vi "Doppler_SVM.vi"(7 "PRF1/2":bool=TRUE, 9 "Doppler Params":T1={"Dopp Filter Order"=2, "Window length"=64, "Window Increment"=64, "Start f"=0.05, "lDoppler cutouff"=10.0, "FFT Length"=512, "SlowTime (Hz)"=100.0} {"Start f" format="%0.3f"; "SlowTime (Hz)" format="%0.1f"; "lDoppler cutouff" format="%0.3f"}, 10 "Input Array":csg[][][](array[numeric]), 11 "Header In":T4={"header info"={"Header"="", "Head length"=0}, "A/D info"={"# rf points per line"=0, "# lines per scan"=0, "sample rate MHz"=0, "# A/D bits"=0, "# bytes per A/D"=0, "TGC Flag"=0, "A/D Type"=""}, "Tranducer Info"={"bandwidth"=0.0, "center freq"=0.0, "start freq"=0.0, "ID"=0}, "Scan Info"={"delay"=0.0, "pivot distance"=0.0, "sector scan angle"=0.0, "operator"="", "Scan Mode"="", "location"=""}, "Time/Date Info"={"date"="", "time"=""}, "RF Info"={"RF file name"="", "RF file att"="", "RF cal file name"="", "RF cal file att"=""}, "Patient Info"={"ID"="", "extended ID"="", "age"=0, "sex"="", "previously\nscanned"="", "PSA"=0.0, "LOS"=1, "Ethnicty 2"=3, "Race"=3}, "Tissue Type"={"organ"=0, "disease type"=0, "disease location"=0, "IQ_pts"=0, "RcvBuffer"=0, "RcvFrame"=0, "IQBuff"=0, "IQFrame"=0, "IQPage"=0}, "Votage scaling"={"Digitizer (dB)"=0.0, "Gain (dB)"=0.0, "Atten (dB)"=0.0}, "Comment"="", "Misc Info"={"avg num"=0, "c speed"=0, "Div By or SF zones"=0, "XMIT CHS"=0, "RCV CHS"=0, "Xmit angle"=0.0}, "Therapy Parameters"={"Theraputic Freq (MHz)"=0.1, "Time on (s)"=1.0, "Therapy amplitude (mV)"=50.0, "Lines Before"=20, "Lines After"=80}, "Scan Settings"={"Energy (uJ or V)"=0, "Damp (Ohm) or Fc"=0, "HP Filt (KHz)"=0, "LP Filt (MHz)"=0, "Gain (db)"=0, "prf (kHz)"=0.0, "Distance between\nscan lines (um)"=0, "Distance between\nscan planes (um)"=0, "Scan line gap (um)"=0.0, "Scan plane gap (um)"=0.0}, "Compression Parameters"={"F1 (MHz)"=0.0, "F2 (MHz)"=0.0, "% taper"=0.0, "duration"=0.0}, "Patient Info Xtra"={"First Name"="", "Last Name"="", "Notes"=""}, "ROI Box"=[]} {"Compression Parameters"."% taper" min=50 max=1000 format="%.2f"; "Compression Parameters"."F2 (MHz)" format="%.3f"; "Compression Parameters"."F1 (MHz)" format="%.3f"; "Scan Settings"."prf (kHz)" format="%.2f"; "Therapy Parameters"."Therapy amplitude (mV)" min=50 max=1000 format="%.2f"; "Therapy Parameters"."Time on (s)" format="%.3f"; "Therapy Parameters"."Theraputic Freq (MHz)" format="%.3f"; "Patient Info"."Race" items=["Am Ind or Alaska", "Asian", "Hawaiian, Pac Isl", "Black or Afr Amer", "White", "more than one race", "unknown"]; "Patient Info"."Ethnicty 2" items=["Hispanic", "Non-Hispanic", "unknown"]; "Patient Info"."LOS" items=["1", "2", "3", "4", "5"]; "Patient Info"."PSA" format="%.1f"; "Scan Info"."delay" format="%.2f"; "Scan Info"."pivot distance" format="%.2f"; "Scan Info"."sector scan angle" format="%.2f"; "Tranducer Info"."bandwidth" format="%.2f"; "Tranducer Info"."center freq" format="%.2f"; "Tranducer Info"."start freq" format="%.2f"}) -> (2 "output cluster":T3, 3 "Filtered Output":cdb[][][](array[numeric]))   [LabVIEW 2022 SP3]
uses:
  ViewData/-ReadEye/Header.ctl
  <vilib>/Analysis/Matrix/Datatypes/ComplexMatrix.ctl
  DopplerParams.ctl
  <vilib>/Analysis/7linalg.llb/Complex Conjugate Transpose Matrix.vi
  <vilib>/Analysis/baseanly.llb/Complex A x B.vi
  <vilib>/Analysis/7linalg.llb/Complex Eigenvalues and Vectors.vi
  <vilib>/Analysis/4window.llb/Hamming Window (CDB).vi
  <vilib>/Analysis/2dsp.llb/Complex FFT.vi
  <vilib>/Analysis/baseanly.llb/Scale 1D.vi
  <vilib>/Analysis/4window.llb/AllCosWindow (CDB).vi
  <vilib>/Analysis/NI_AALPro.lvlib
  <vilib>/Analysis/NI_AALBase.lvlib
  <vilib>/Analysis/Matrix/NI_Matrix.lvlib
panel:
  out "Spectro fig":dbl[][](graph)
  out "Sing Value Sum":dbl[](graph)
  out "raw":sgl[][](graph)
  out "Dop Freq":dbl[](graph)
  out "filtered data":dbl[][](graph)
  in  "v? or f":bool
  out "Covariance":dbl[][](graph)
  out "Sing Value Diff Ratio":dbl[](graph)
  out "Sing Values":dbl[](graph)
  in  "GapCutOff":i16
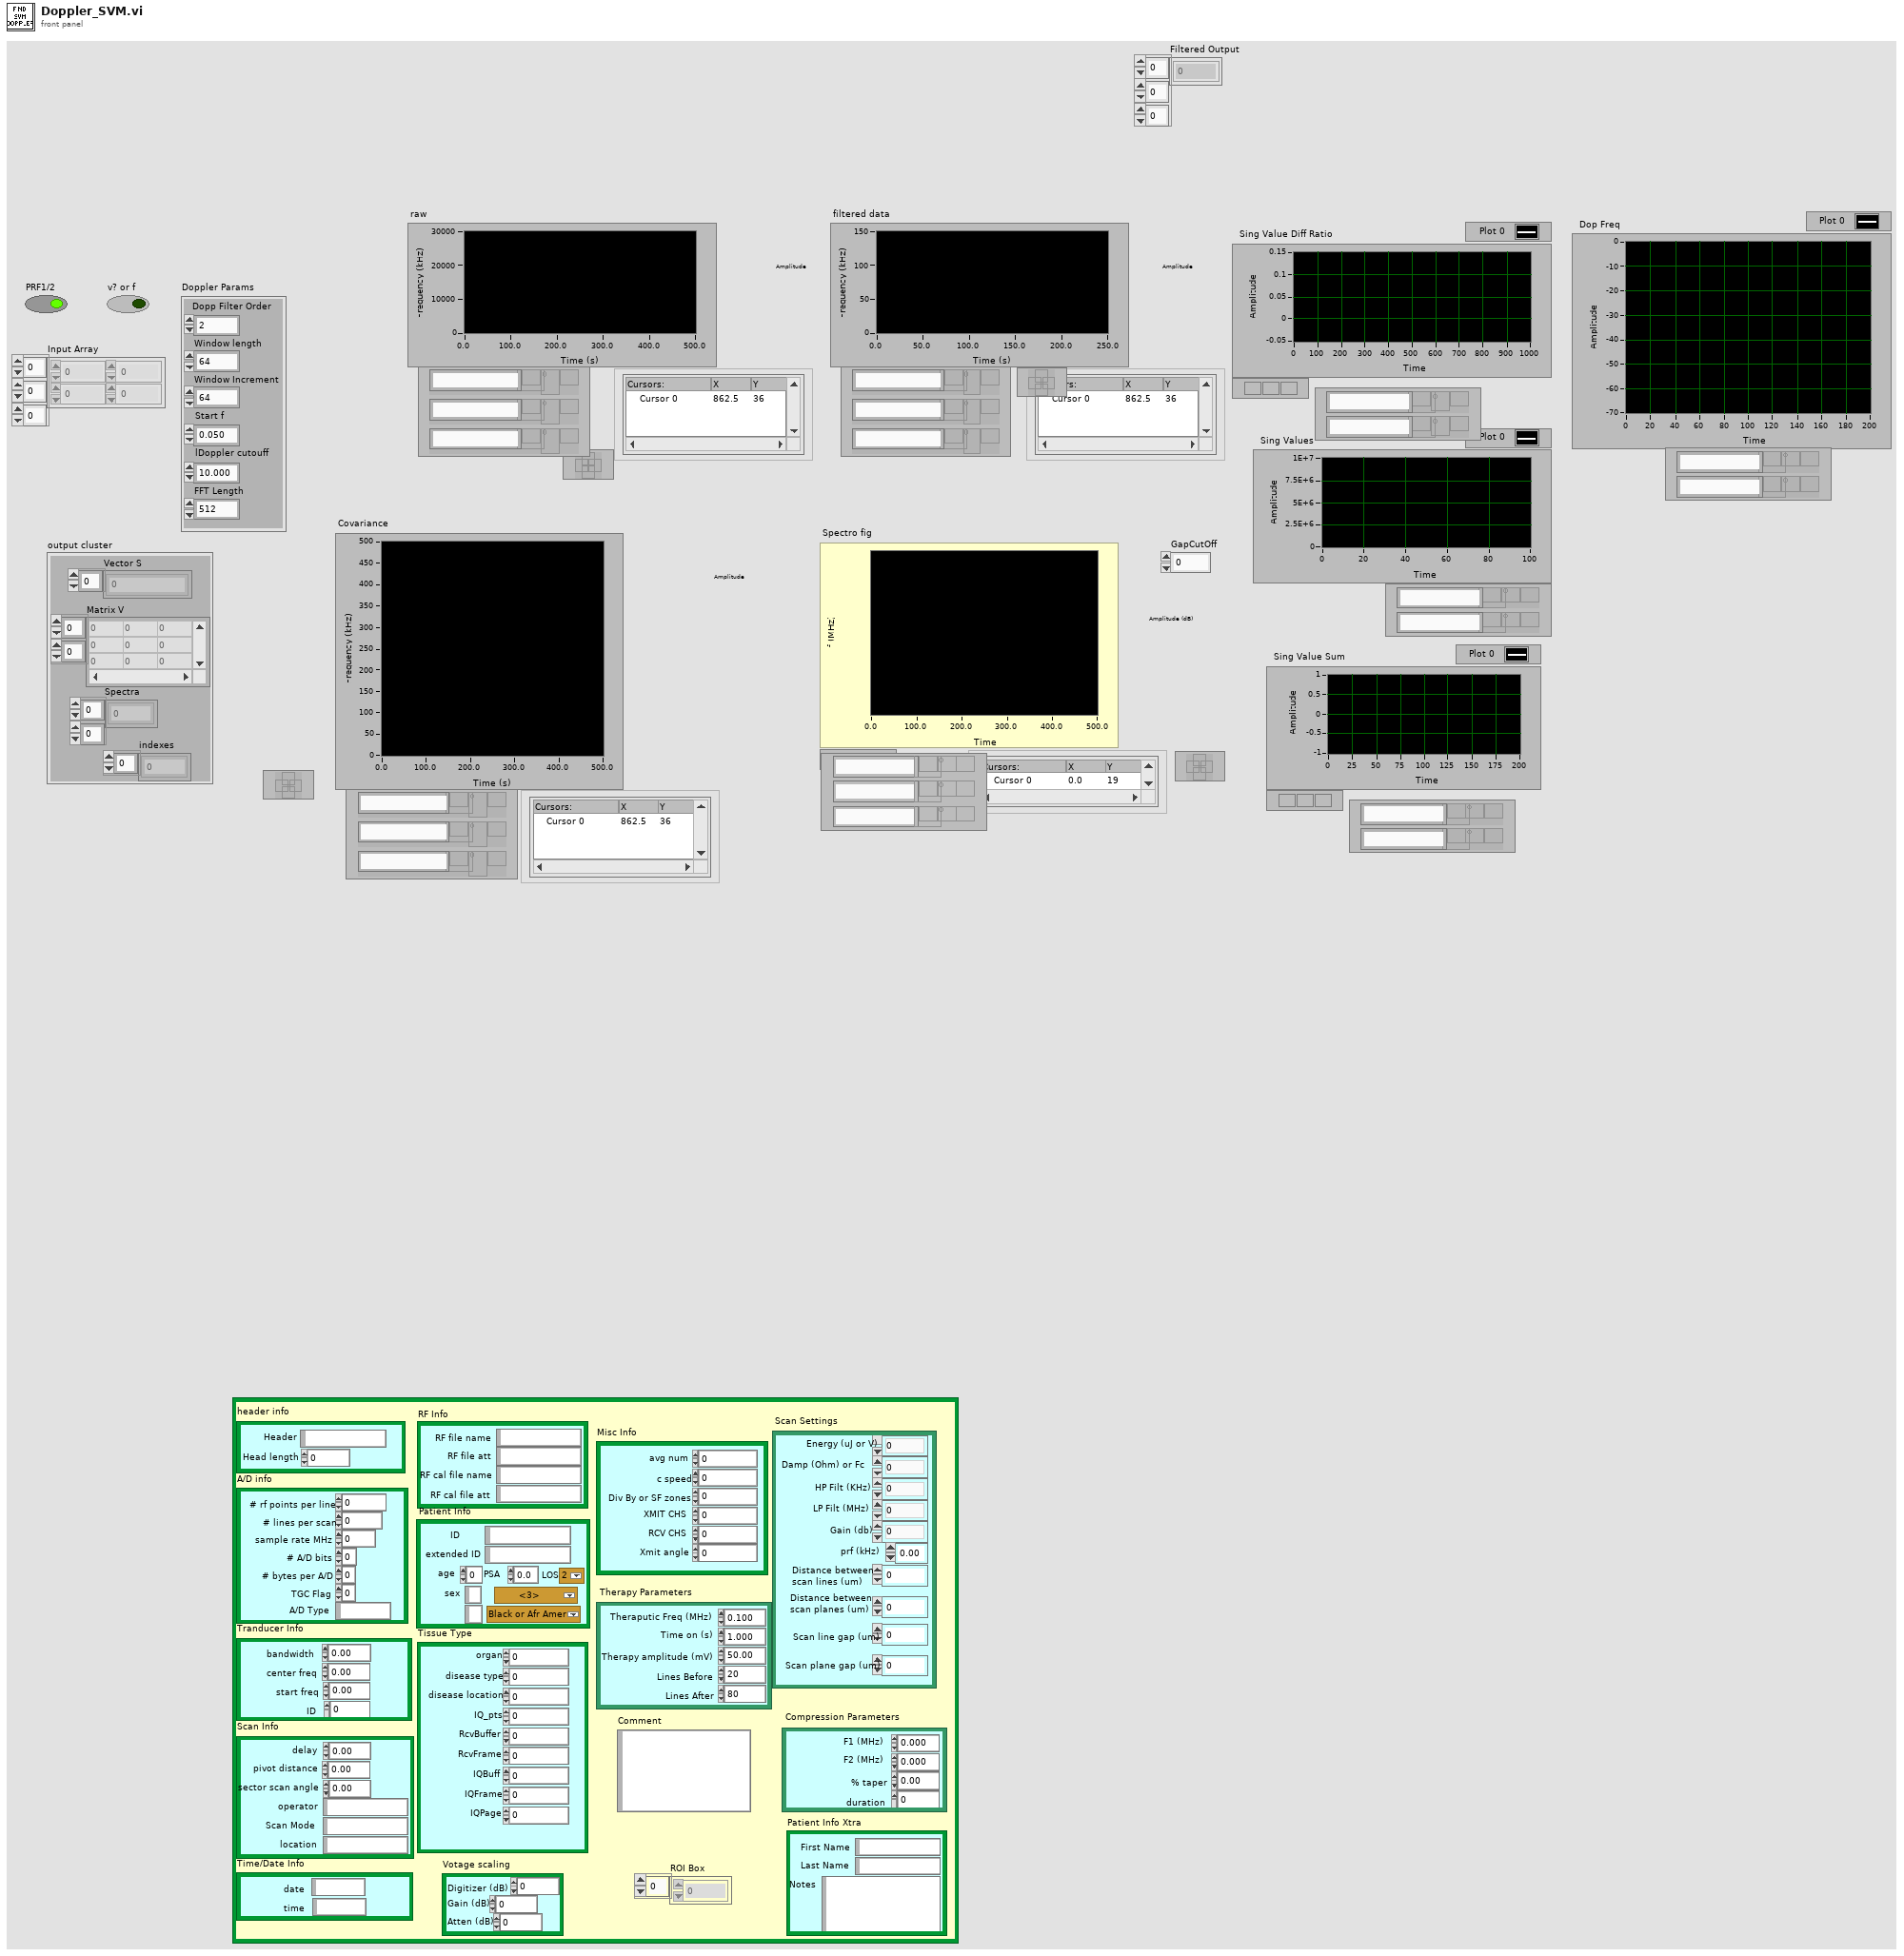
[diagram p1: front panel]
types:
  T1 = typedef "DopplerParams.ctl" = cluster{"Dopp Filter Order":i32, "Window length":i32, "Window Increment":i32, "Start f":dbl, "lDoppler cutouff":dbl, "FFT Length":i32, "SlowTime (Hz)":dbl}
  T2 = typedef "NI_Matrix.lvlib/ComplexMatrix.ctl" = cdb[][]
  T3 = cluster{"Vector S":cdb[], "Matrix V":T2, "Spectra":dbl[][], "indexes":i32[]}
  T4 = typedef "Header.ctl" = cluster{"header info":cluster{"Header":string, "Head length":i16}, "A/D info":cluster{"# rf points per line":u16, "# lines per scan":u16, "sample rate MHz":u16, "# A/D bits":i16, "# bytes per A/D":u16, "TGC Flag":u16, "A/D Type":string}, "Tranducer Info":cluster{"bandwidth":sgl, "center freq":sgl, "start freq":sgl, "ID":i32}, "Scan Info":cluster{"delay":sgl, "pivot distance":sgl, "sector scan angle":sgl, "operator":string, "Scan Mode":string, "location":string}, "Time/Date Info":cluster{"date":string, "time":string}, "RF Info":cluster{"RF file name":string, "RF file att":string, "RF cal file name":string, "RF cal file att":string}, "Patient Info":cluster{"ID":string, "extended ID":string, "age":u16, "sex":string, "previously\nscanned":string, "PSA":sgl, "LOS":u8, "Ethnicty 2":u8, "Race":u8}, "Tissue Type":cluster{"organ":i16, "disease type":i16, "disease location":i16, "IQ_pts":u16, "RcvBuffer":u8, "RcvFrame":u16, "IQBuff":u8, "IQFrame":u16, "IQPage":u8}, "Votage scaling":cluster{"Digitizer (dB)":sgl, "Gain (dB)":sgl, "Atten (dB)":sgl}, "Comment":string, "Misc Info":cluster{"avg num":u16, "c speed":i16, "Div By or SF zones":i16, "XMIT CHS":u8, "RCV CHS":u8, "Xmit angle":sgl}, "Therapy Parameters":cluster{"Theraputic Freq (MHz)":sgl, "Time on (s)":sgl, "Therapy amplitude (mV)":sgl, "Lines Before":u16, "Lines After":u16}, "Scan Settings":cluster{"Energy (uJ or V)":u8, "Damp (Ohm) or Fc":u8, "HP Filt (KHz)":u8, "LP Filt (MHz)":u8, "Gain (db)":u8, "prf (kHz)":sgl, "Distance between\nscan lines (um)":u16, "Distance between\nscan planes (um)":u16, "Scan line gap (um)":sgl, "Scan plane gap (um)":sgl}, "Compression Parameters":cluster{"F1 (MHz)":sgl, "F2 (MHz)":sgl, "% taper":sgl, "duration":sgl}, "Patient Info Xtra":cluster{"First Name":string, "Last Name":string, "Notes":string}, "ROI Box":u16[]}
  T5 = cluster{"Y Scale Mult":dbl, "Y Scale offset":dbl, "X Scale Mult":dbl, "Dop F offset":dbl, "Dop interval":dbl}
  T6 = cluster{"Eigenvalues":cdb[], "Eigenvectors":T2, dbl[][], i32[]}
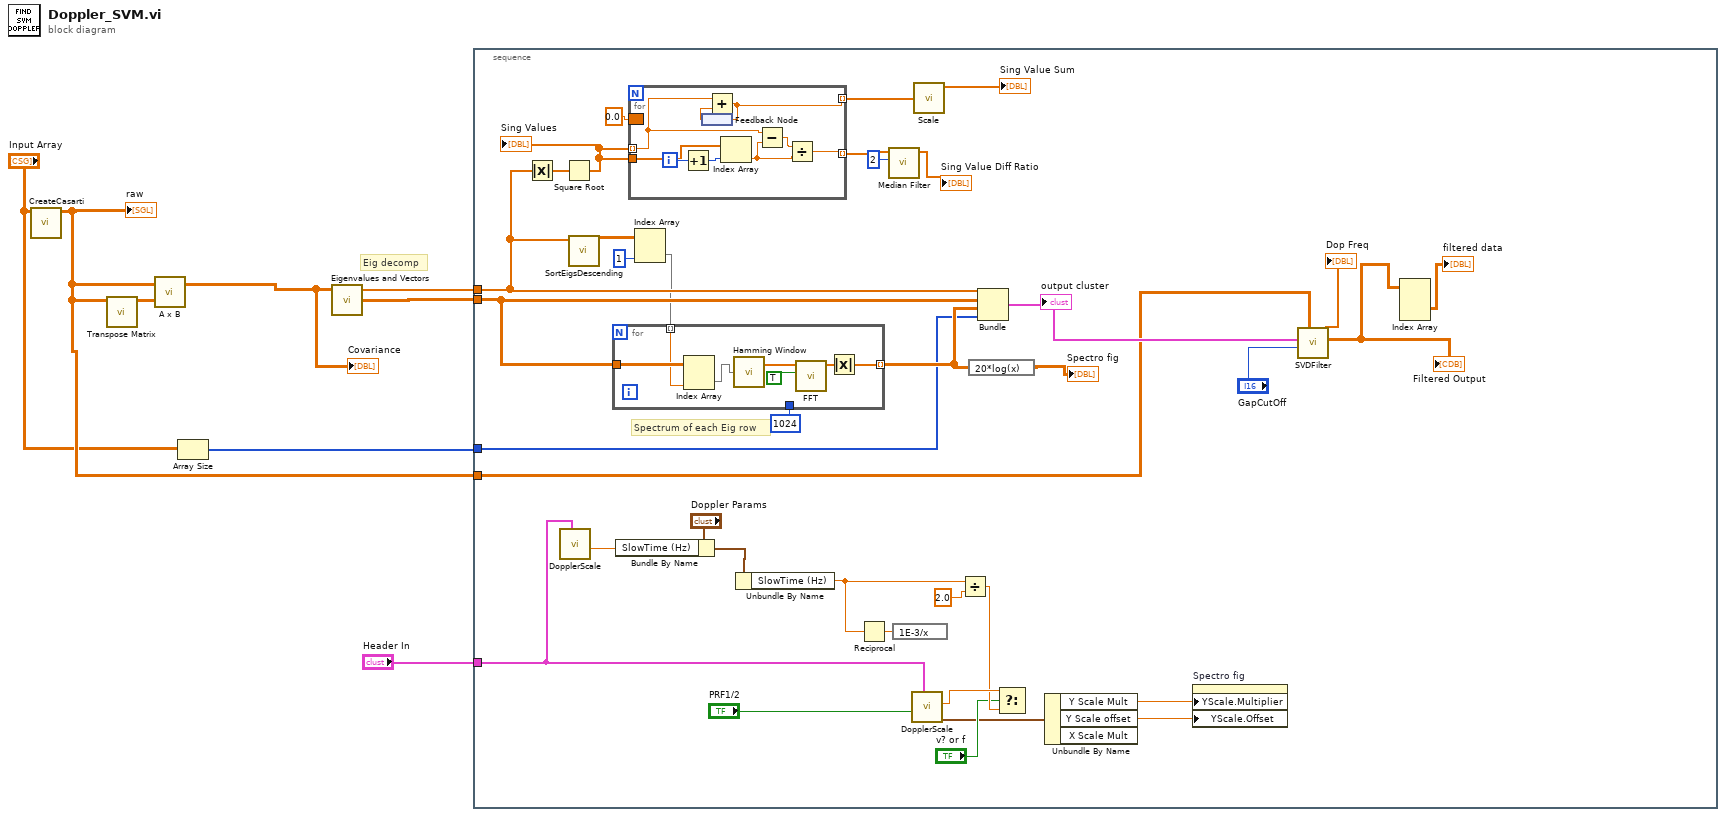
[diagram p0: block diagram]
diagram:
  # "Eig decomp"
  n1 = call "CreateCasarti.vi"("Input Array"="Input Array") -> ("output array"=w5:csg[][])  [unwired: 10 in]
  "raw" <- w5
  n2 = call-poly <vilib>:"Transpose Matrix.vi"("Input Matrix"=w5) -> ("Matrix Conjugate Transpose"=w6:T2)  [unwired: 9 in, 1 out]
  n3 = call-poly <vilib>:"A x B.vi"("B"=w6, "A"=w5) -> ("A x B"=w2:T2)  [unwired: 1 out]
  "Covariance" <- w2
  n4 = Array Size(array="Input Array") -> (size(s)=w3:i32[])
  n5 = call-poly <vilib>:"Eigenvalues and Vectors.vi"("Input Matrix"=w2) -> ("Eigenvectors"=w1:T2, "Eigenvalues"=w8:cdb[])  [unwired: 2 in, 1 out]
  n6 = stacked-sequence {
    tunnel: w8 -> [w14]
    tunnel: w1 -> [w11]
    tunnel: "Header In" -> [w29]
    tunnel: w5 -> [w19]
    tunnel: w3 -> [w18]
    frame #0 {
      # "Spectrum of each Eig row"
      n7 = Absolute Value(x=w14) -> (abs(x)=w15:dbl[])
      n8 = call "DopplerScale.vi"("Header In"=w29) -> ("slow-time sampling"=w27:dbl)  [unwired: 7 in, 3 out]
      n9 = Square Root(x=w15) -> (sqrt(x)=w33:dbl[])
      "Sing Values" <- w33
      n10 = call "SortEigsDescending.vi"("Array in"=w14) -> ("Array out"=w13:dbl[][])  [unwired: 10 in]
      n11 = Bundle By Name(cluster="Doppler Params", "SlowTime (Hz)"=w27) -> (w26:T1)
      n12 = for {
        tunnel: w33 -> [w53]
        tunnel: w33 -> [w49] mode=indexing
        tunnel: [w48] -> w23 mode=indexing
        tunnel: [w50] -> w24 mode=indexing
        border: 0.0 -> [_]
        i -> [w54]
        n13 = Increment(x=w54) -> (x+1=w52:i32)
        n14 = feedback #1() -> (w51:dbl)
        n15 = Add(x=w49, y=w51) -> (x+y=w50:dbl)
        n16 = feedback-in #1(w50) -> ()
        n17 = Index Array(array=w53, index=w52) -> (element=w47:dbl)
        n18 = Subtract(x=w49, y=w47) -> (x-y=w46:dbl)
        n19 = Divide(x=w46, y=w47) -> (x/y=w48:dbl)
      }
      n20 = Index Array(array=w13, index (col)=1 ("disabled index (col)")) -> (element=w10:dbl[])  [unwired: 1 in]
      n21 = for {
        tunnel: w11 -> [w58]
        tunnel: [w59] -> w20 mode=indexing
        tunnel: 1024 ("FFT size") -> [_]
        tunnel: w10 -> [w57] mode=indexing
        n22 = Index Array(array=w58, index (col)=w57) -> (element=w56:cdb[])  [unwired: 1 in]
        n23 = call-poly <vilib>:"Hamming Window.vi"("X"=w56) -> ("Windowed X"=w55:cdb[])  [unwired: 1 out]
        n24 = call-poly <vilib>:"FFT.vi"("shift?"=TRUE, "X"=w55) -> ("FFT {X}"=w61:cdb[])  [unwired: 8 in, 1 out]
        n25 = Absolute Value(x=w61) -> (abs(x)=w59:dbl[])
      }
      n26 = Unbundle By Name(w26) -> ("SlowTime (Hz)"=w31:dbl)
      n27 = Reciprocal(x=w31) -> (1/x=w45:dbl)
      n28 = call <vilib>:"Median Filter.vi"("left rank"=2, "X"=w23) -> ("Filtered X"=→"Sing Value Diff Ratio":dbl[])  [unwired: 8 in, 1 out]
      n29 = expression code="1E-3/x"(w45) -> ()  [unwired: 1 out]
      n30 = call "DopplerScale.vi"("Header In"=w29, "PRF1/2"="PRF1/2") -> ("output cluster"=w40:T5, "max doppler velocity cm/s"=w43:dbl)  [unwired: 6 in, 2 out]
      n31 = call-poly <vilib>:"Scale.vi"("X"=w24) -> ("Y=(X-offset)/scale"=→"Sing Value Sum":dbl[])  [unwired: 3 out]
      n32 = Divide(x=w31, y=2.0) -> (x/y=w42:dbl)
      n33 = expression code="20*log(x)"(w20) -> (→"Spectro fig":dbl[][])
      n34 = Bundle("Eigenvalues"=w14, "Eigenvectors"=w11, w20, w18) -> (w37:T6)  [unwired: 1 in]
      "output cluster" <- w37
      n35 = Select(t=w43, s="v? or f", f=w42) -> ()  [unwired: 1 out]
      n36 = Unbundle By Name(w40) -> ("Y Scale Mult"=w39:dbl, "Y Scale offset"=w38:dbl)  [unwired: 1 out]
      n37 = property on="Spectro fig" class="IntGraph (strict)"("YScale.Multiplier"=w39, "YScale.Offset"=w38) -> ()  [unwired: 2 in, 2 out]
      n38 = call "SVDFilter.vi"("Input Image"=w19, "Low zero index"="GapCutOff", "output cluster"=w37) -> ("Filtered Output"=w17:cdb[][][], "log singular"=→"Dop Freq":dbl[])  [unwired: 7 in]
      "Filtered Output" <- w17
      n39 = Index Array(array=w17) -> (element=→"filtered data":cdb[][])  [unwired: 3 in]
    }
  }
